vi "HP_Butter.vi"(1 "low cutoff freq: fl":dbl, 2 "Samping Frequency":dbl, 3 "Signal Sequence":dbl[](array[numeric])) -> (0 "Array":dbl[](array[numeric]))   [LabVIEW 2019]
uses:
  <vilib>/Analysis/3filter.llb/Filter Passband Type.ctl
  <vilib>/Analysis/3filter.llb/Butterworth Filter (DBL).vi
  <vilib>/Analysis/NI_AALBase.lvlib
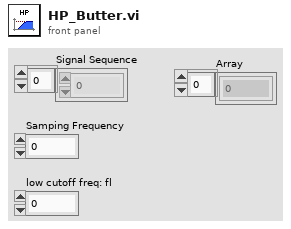
[diagram p1: front panel]
types:
  T1 = typedef "NI_AALBase.lvlib/Filter Passband Type.ctl" = enum32{"Lowpass", "Highpass", "Bandpass", "Bandstop"}
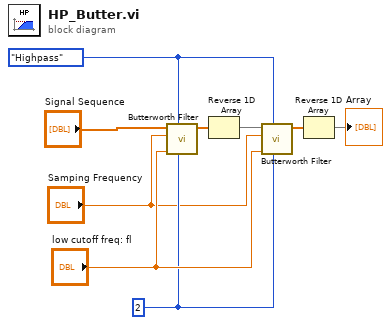
[diagram p0: block diagram]
diagram:
  w1 = Filter_Passband_Type."Highpass" ("filter type")
  w7 = 2 ("order")
  n1 = call-poly <vilib>:"Butterworth Filter.vi"("order"=w7, "filter type"=w1, "low cutoff freq: fl"="low cutoff freq: fl", "sampling freq: fs"="Samping Frequency", "X"="Signal Sequence") -> ("Filtered X"=w2:dbl[])  [unwired: 3 in, 1 out]
  n2 = Reverse 1D Array(array=w2) -> (reversed array=w3:dbl[])
  n3 = call-poly <vilib>:"Butterworth Filter.vi"("order"=w7, "filter type"=w1, "low cutoff freq: fl"="low cutoff freq: fl", "sampling freq: fs"="Samping Frequency", "X"=w3) -> ("Filtered X"=w4:dbl[])  [unwired: 3 in, 1 out]
  n4 = Reverse 1D Array(array=w4) -> (reversed array=→"Array":dbl[])
